vi "Initialize VIs Stream.vi"(8 "error in (no error)":errorcluster, 11 "Channel in":refnum<class "Channel.lvclass">) -> (0 "error out":errorcluster, 3 "Channel out":refnum<class "Channel.lvclass">)   [LabVIEW 2018, in "Channel.lvclass"]
uses:
  Channel.lvclass
  Channel.lvclass/Channel.ctl
  Save Image/Save Image.lvclass/Save Image.ctl
  Save Image/Save Image.lvclass
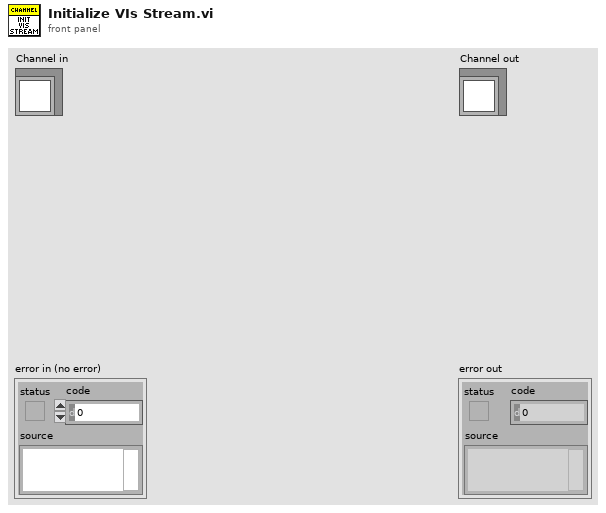
[diagram p1: front panel]
types:
  T1 = cluster{"COMNENT":string, "OBSTYPE":string, "ACSVRSN":string, "CHANNEL":u16, "LAST_IMG_NAME":string, "NIGHTDIR":string}
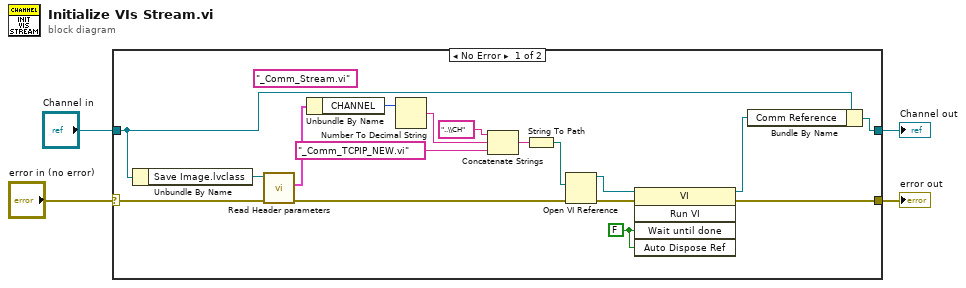
[diagram p0: block diagram]
diagram:
  n1 = case shown="No Error" "error in (no error)" {
    selector: "error in (no error)" -> [w9 w23]
    tunnel: [w6 w23] -> w3
    tunnel: [w19 w22] -> w1
    tunnel: "Channel in" -> [w15 w22]
    frame No Error {
      (unwired) "_Comm_Stream.vi" ("name or relative path")
      w20 = FALSE ("Wait Until Done")
      n2 = Unbundle By Name(w15) -> ("Save Image.lvclass"=w14:refnum<class "Save Image.lvclass">)
      n3 = call "Read Header parameters.vi"("error in (no error)"=w9, "Save Image in"=w14) -> ("error out"=w13:errorcluster, "Header parameters"=w12:T1)  [unwired: 7 in, 1 out]
      n4 = Unbundle By Name(w12) -> ("CHANNEL"=w11:u16)
      n5 = Number To Decimal String(number=w11) -> (decimal integer string=w7:string)  [unwired: 1 in]
      n6 = Concatenate Strings("..\\CH" ("name or relative path"), w7, "_Comm_TCPIP_NEW.vi" ("name or relative path")) -> (w17:string)
      n7 = String To Path(string=w17) -> (path=w18:path)
      n8 = Open VI Reference(vi path=w18, error in (no error)=w13) -> (vi reference=w21:refnum<vi>, error out=w16:errorcluster)  [unwired: 4 in]
      n9 = invoke class="VI" method="Run VI"(reference=w21, error in=w16, "Wait until done"=w20, "Auto Dispose Ref"=w20) -> (reference out=w10:refnum<vi>, error out=w6:errorcluster)  [unwired: 1 in, 3 out]
      n10 = Bundle By Name(cluster=w15, "Comm Reference"=w10) -> (w19:refnum<class "Channel.lvclass">)
    }
    frame Error {
    }
  }
  "error out" <- w3
  "Channel out" <- w1
